vi "server 1.vi"() -> ()   [LabVIEW 2018]
doc: "This is the TCP server VI that supports multiple connections from client VIs."
uses:
  controls/TCP Multiple Connections State.ctl
  controls/TCP Multiple Connections Data.ctl
panel:
  out "Client IP":string
  out "color box":u32(colorbox)
  in  "Stop":bool
  out "Sent Data":dbl
  out "# of Connections":i32
  # "6341"
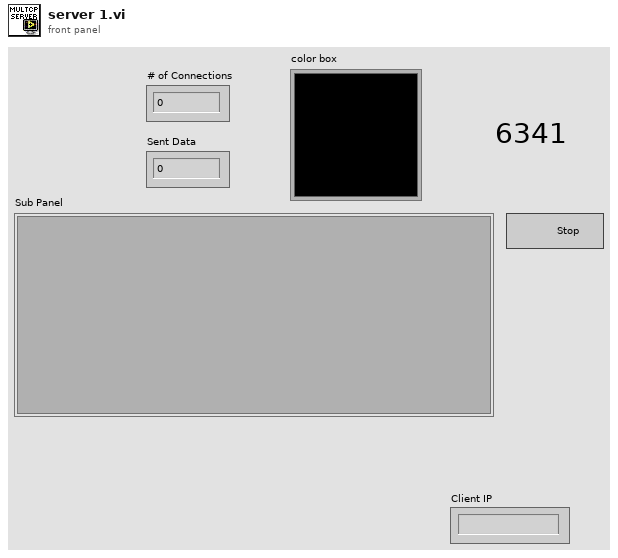
[diagram p1: front panel]
types:
  T1 = typedef "TCP Multiple Connections Data.ctl" = cluster{"Clients":refnum<k5>[], "Listener":refnum<k5>}
  T2 = typedef "TCP Multiple Connections State.ctl" = enum16{"Initialize", "Status Check", "Send Data", "Stop"}
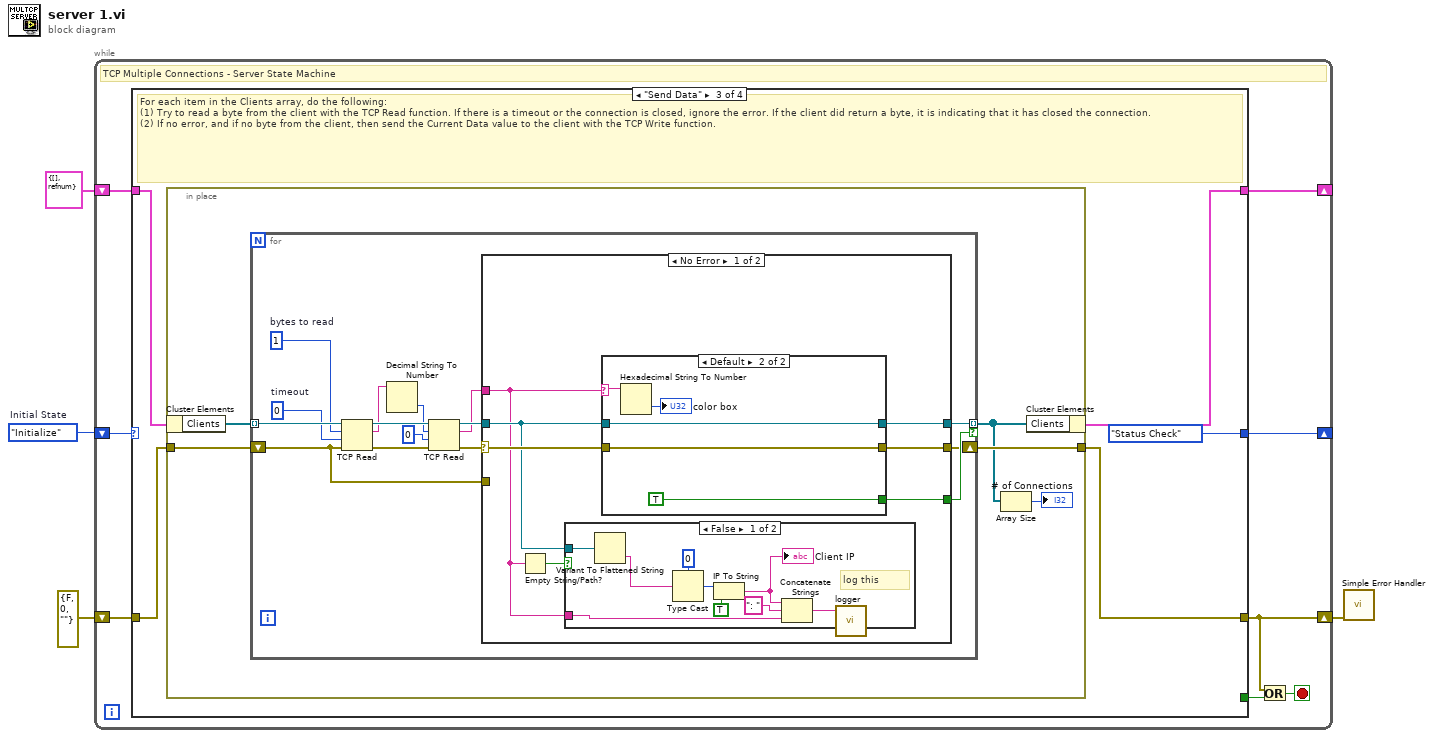
[diagram p0: block diagram]
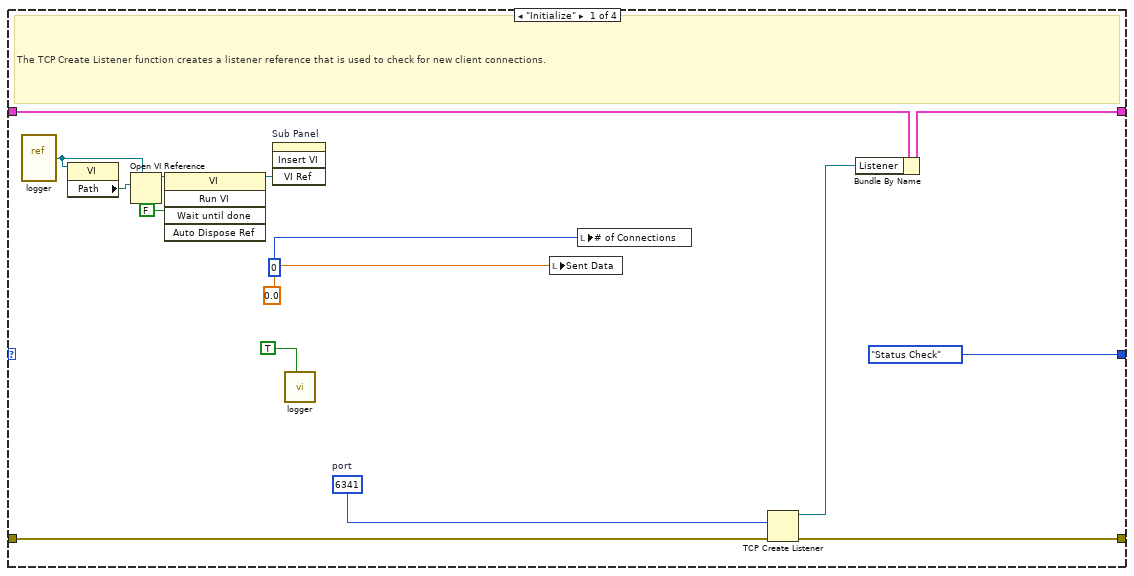
[diagram p2: hidden frame]
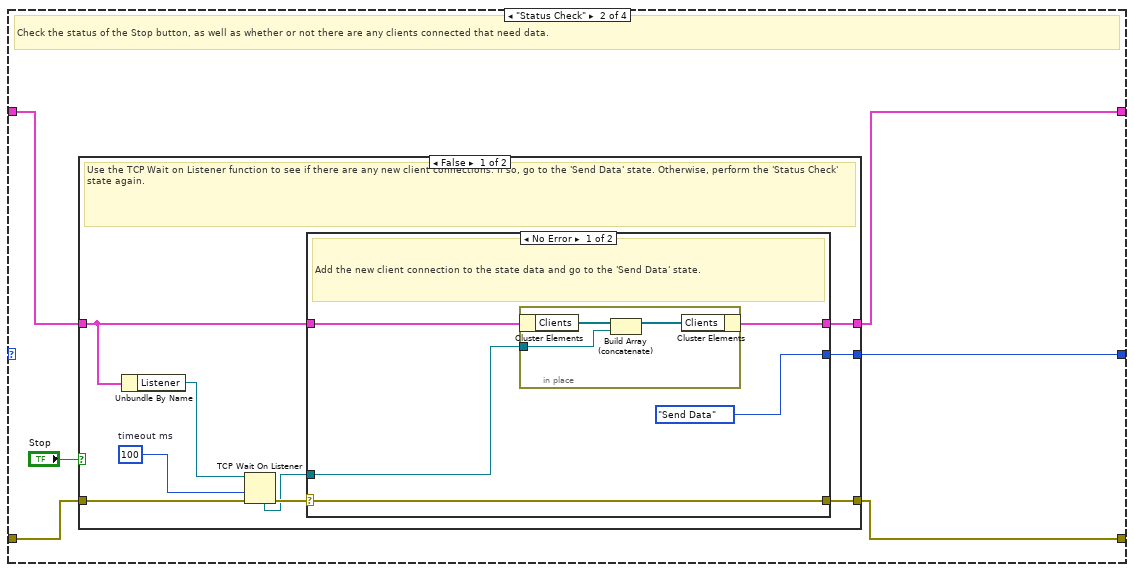
[diagram p3: hidden frame]
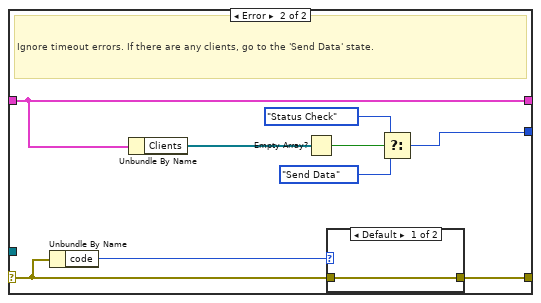
[diagram p4: hidden frame]
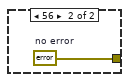
[diagram p5: hidden frame]
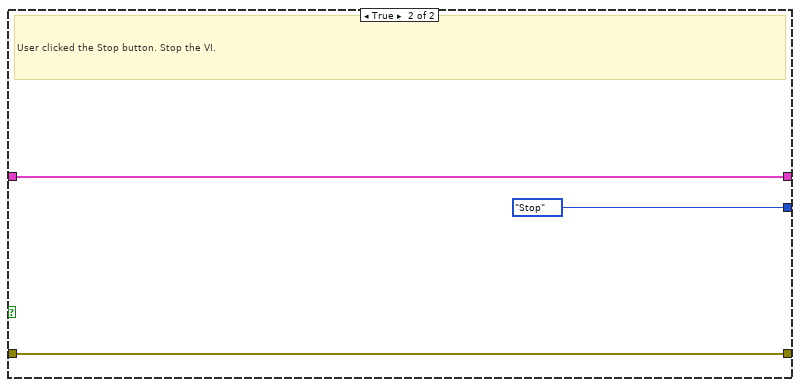
[diagram p6: hidden frame]
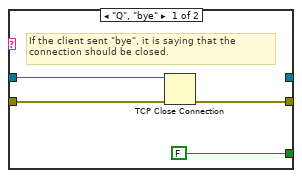
[diagram p8: hidden frame]
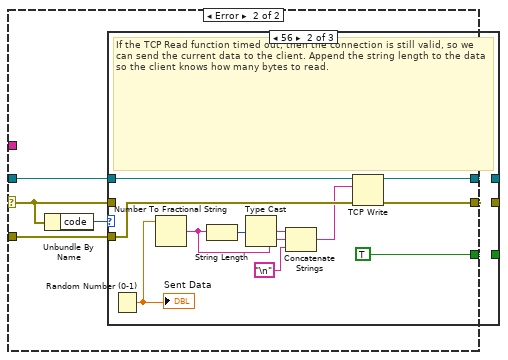
[diagram p9: hidden frame]
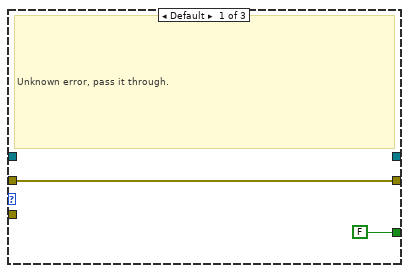
[diagram p10: hidden frame]
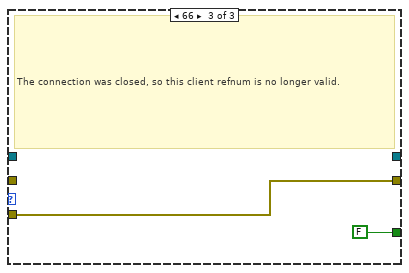
[diagram p11: hidden frame]
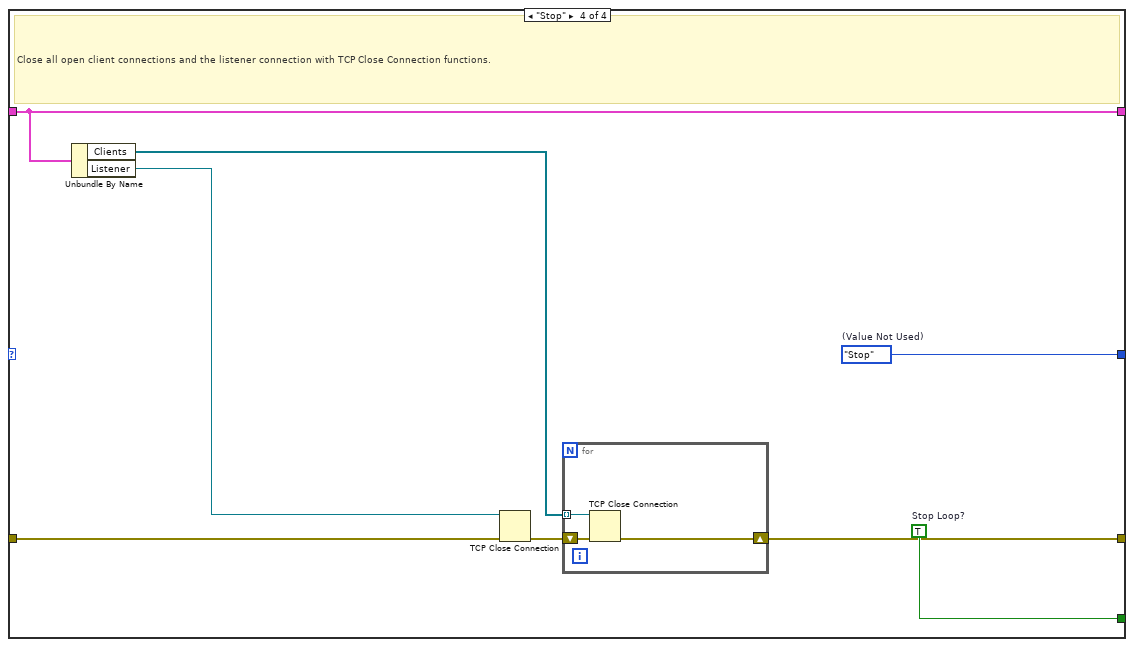
[diagram p12: hidden frame]
diagram:
  w4 = TCP_Multiple_Connections_State."Initialize"  # Initial State
  n1 = while {
    shift-right: [w11] -> _
    shift-left: w4 -> [w12]
    shift-right: [w9] -> _
    shift-left: T1 {"Clients"=[], "Listener"=refnum} ("Data") -> [w10]
    shift-right: [w5] -> w1
    shift-left: errorcluster {"status"=FALSE, "code"=0, "source"=""} ("error constant") -> [w8]
    stop <- w6 stop-if-true
    # "TCP Multiple Connections - Server State Machine"
    n2 = case shown="\"Send Data\"" w12 {
      tunnel: [TCP_Multiple_Connections_State."Status Check" ("States") w33 TCP_Multiple_Connections_State."Status Check" ("States") w137] -> w11
      tunnel: [_ _ _ w144] -> w7
      tunnel: w10 -> [w25 w31 w67 w143]
      tunnel: [w24 w30 w65 w143] -> w9
      tunnel: w8 -> [w27 w29 w69 w142]
      tunnel: [w26 w28 w68 w140] -> w5
      frame "Initialize" {
        w22 = u16 6341  # port
        # "The TCP Create Listener function creates a listener reference that is used to check for new client connections."
        n3 = vi-ref "logger.vi"() -> (w17:refnum<vi>)
        n4 = property class="VI"(reference=w17) -> ("Path"=w16:path)  [unwired: 1 in, 2 out]
        n5 = Open VI Reference(type specifier VI Refnum (for type only)=w17, vi path=w16) -> (vi reference=w15:refnum<vi>)  [unwired: 4 in, 1 out]
        n6 = invoke class="VI" method="Run VI"(reference=w15, "Wait until done"=FALSE ("Wait Until Done")) -> (reference out=w13:refnum<vi>)  [unwired: 3 in, 4 out]
        n7 = invoke on="Sub Panel" class="SubPnl" method="Insert VI"("VI Ref"=w13) -> ()  [unwired: 3 in, 4 out]
        n8 = call "logger.vi"("reset? (F)"=TRUE) -> ()  [unwired: 8 in, 1 out]
        n9 = local write "Sent Data"(0.0 ("Current Data")) -> ()
        n10 = local write "# of Connections"(0 ("Number of Client Connections")) -> ()
        n11 = TCP Create Listener(8:w27, 10:w22) -> (0:w26:errorcluster, 3:w23:refnum<k5>)  [unwired: 4 out]
        n12 = Bundle By Name(cluster=w25, "Listener"=w23) -> (w24:T1)
      }
      frame "Status Check" {
        # "Check the status of the Stop button, as well as whether or not there are any clients connected that need data."
        n13 = case shown="False" "Stop" {
          tunnel: [w42 TCP_Multiple_Connections_State."Stop" ("States")] -> w33
          tunnel: w29 -> [w41 w64]
          tunnel: [w34 w64] -> w28
          tunnel: w31 -> [w37 w63]
          tunnel: [w36 w63] -> w30
          frame False {
            w40 = 100  # timeout ms
            # "Use the TCP Wait on Listener function to see if there are any new client connections. If so, go to the 'Send Data' state. Otherwise, perform the 'Status Check' state again."
            n14 = Unbundle By Name(w37) -> ("Listener"=w35:refnum<k5>)
            n15 = TCP Wait On Listener(8:w41, 9:w40, 11:w35) -> (0:w39:errorcluster, 4:w38:refnum<k5>)  [unwired: 4 out]
            n16 = case shown="No Error" w39 {
              selector: w39 -> [w45 w59]
              tunnel: [TCP_Multiple_Connections_State."Send Data" ("States") w53] -> w42
              tunnel: w38 -> [w46 _]
              tunnel: w37 -> [w47 w56]
              tunnel: [w44 w56] -> w36
              tunnel: [w45 w57] -> w34
              frame No Error {
                # "Add the new client connection to the state data and go to the 'Send Data' state."
                n17 = in-place {
                  in-place-border: w46 -> [w48]
                  n18 = in-place-cluster #1(w47) -> ("Clients"=w50:refnum<k5>[])
                  n19 = Build Array (concatenate)(w50, w48) -> (w49:refnum<k5>[])
                  n20 = in-place-cluster #1("Clients"=w49) -> (w44:T1)
                }
              }
              frame Error {
                # "Ignore timeout errors. If there are any clients, go to the 'Send Data' state."
                n21 = Unbundle By Name(w59) -> ("code"=w58:i32)
                n22 = Unbundle By Name(w56) -> ("Clients"=w55:refnum<k5>[])
                n23 = Empty Array?(array=w55) -> (empty?=w54:bool)
                n24 = case shown="Default" w58 {
                  tunnel: w59 -> [w60 _]
                  tunnel: [w60 w61] -> w57
                  frame Default {
                  }
                  frame 56 {
                    w61 = errorcluster {"status"=FALSE, "code"=0, "source"=""}  # no error
                  }
                }
                n25 = Select(t=TCP_Multiple_Connections_State."Status Check" ("States"), s=w54, f=TCP_Multiple_Connections_State."Send Data" ("States")) -> (s? t:f=w53:T2)
              }
            }
          }
          frame True {
            # "User clicked the Stop button. Stop the VI."
          }
        }
      }
      frame "Send Data" {
        # "For each item in the Clients array, do the following:\n(1) Try to read a byte from the client with the TCP Read function. If there is a timeout or the connection is closed, ignore the error. If the client did return a byte, it is indicating that it has closed the connection.\n(2) If no error, and if no byte from the client, then send the Current Data value to the client with the TCP Write function."
        n26 = in-place {
          in-place-border: w69 -> [w74]
          in-place-border: [w73] -> w68
          n27 = in-place-cluster #2(w67) -> ("Clients"=w71:refnum<k5>[])
          n28 = for {
            tunnel: w71 -> [w89] mode=indexing
            shift-right: [w84] -> w73
            shift-left: w74 -> [w83]
            tunnel: [w86] -> w70 mode=indexing if=w85
            w87 = 0  # timeout
            w88 = 1  # bytes to read
            n29 = TCP Read(connection ID=w89, bytes to read=w88, error in (no error)=w83, 9:w87) -> (connection ID out=w82:refnum<k5>, data out=w80:string, error out=w78:errorcluster)  [unwired: 1 out]
            n30 = Decimal String To Number(string=w80) -> (number=w81:i32)  [unwired: 2 in, 1 out]
            n31 = TCP Read(connection ID=w82, bytes to read=w81, error in (no error)=w78, 9:0 ("timeout ms (25000)")) -> (connection ID out=w79:refnum<k5>, data out=w75:string, error out=w77:errorcluster)  [unwired: 1 out]
            n32 = case shown="No Error" w77 {
              selector: w77 -> [w96 w120]
              tunnel: w79 -> [w91 w117]
              tunnel: w75 -> [w90 _]
              tunnel: [w93 w115] -> w86
              tunnel: [w95 w116] -> w85
              tunnel: [w94 w119] -> w84
              tunnel: w83 -> [_ w118]
              frame No Error {
                # "If the client sent data, it is saying that the connection should be closed."
                n33 = Empty String/Path?(string/path=w90) -> (empty?=w92:bool)
                n34 = case shown="False" w92 {
                  tunnel: w91 -> [w98 _]
                  tunnel: w90 -> [w97 _]
                  frame False {
                    # "log this"
                    n35 = Variant To Flattened String(Variant=w98) -> (data string=w102:string)  [unwired: 1 out]
                    n36 = Type Cast(type=u32 0, x=w102) -> (*(type *) &x=w103:u32)
                    n37 = IP To String(1:TRUE ("dot notation? (F)"), 2:w103) -> (0:w104:string)
                    "Client IP" <- w104
                    n38 = Concatenate Strings(w104, ": " ("string"), w97) -> (w105:string)
                    n39 = call "logger.vi"("new data"=w105) -> ()  [unwired: 8 in, 1 out]
                  }
                  frame True {
                  }
                }
                n40 = case shown="Default" w90 {
                  selector: w90 -> [_ w112]
                  tunnel: w91 -> [w109 w110]
                  tunnel: w96 -> [w108 w114]
                  tunnel: [FALSE TRUE] -> w95
                  tunnel: [w106 w114] -> w94
                  tunnel: [_ w110] -> w93
                  frame "Q", "bye" {
                    # "If the client sent \"bye\", it is saying that the connection should be closed."
                    n41 = TCP Close Connection(connection ID=w109, error in (no error)=w108) -> (error out=w106:errorcluster)  [unwired: 2 out]
                  }
                  frame Default {
                    n42 = Hexadecimal String To Number(string=w112) -> (number=→"color box":u32)  [unwired: 2 in, 1 out]
                  }
                }
              }
              frame Error {
                # "Ignore connection closed and timeout errors"
                n43 = Unbundle By Name(w120) -> ("code"=w121:i32)
                n44 = case shown="56" w121 {
                  tunnel: w120 -> [w123 _ _]
                  tunnel: [w123 w134 w136] -> w119
                  tunnel: w118 -> [_ w130 w136]
                  tunnel: w117 -> [_ w133 _]
                  tunnel: [FALSE TRUE FALSE] -> w116
                  tunnel: [_ w132 _] -> w115
                  frame Default {
                    # "Unknown error, pass it through."
                  }
                  frame 56 {
                    # "If the TCP Read function timed out, then the connection is still valid, so we can send the current data to the client. Append the string length to the data so the client knows how many bytes to read."
                    n45 = Random Number (0-1)() -> (number: 0 to 1=w129:dbl)
                    "Sent Data" <- w129
                    n46 = Number To Fractional String(number=w129) -> (F-format string=w126:string)  [unwired: 3 in]
                    n47 = String Length(string=w126) -> (length=w127:i32)
                    n48 = Type Cast(x=w127) -> (*(type *) &x=w128:string)  [unwired: 1 in]
                    n49 = Concatenate Strings(w128, w126, "\n") -> (w125:string)
                    n50 = TCP Write(connection ID=w133, data in=w125, error in (no error)=w130) -> (connection ID out=w132:refnum<k5>, error out=w134:errorcluster)  [unwired: 2 out]
                  }
                  frame 66 {
                    # "The connection was closed, so this client refnum is no longer valid."
                  }
                }
              }
            }
          }
          n51 = Array Size(array=w70) -> (size(s)=→"# of Connections":i32)
          n52 = in-place-cluster #2("Clients"=w70) -> (w65:T1)
        }
      }
      frame "Stop" {
        w137 = TCP_Multiple_Connections_State."Stop"  # (Value Not Used)
        w144 = TRUE  # Stop Loop?
        # "Close all open client connections and the listener connection with TCP Close Connection functions."
        n53 = Unbundle By Name(w143) -> ("Clients"=w141:refnum<k5>[], "Listener"=w138:refnum<k5>)
        n54 = TCP Close Connection(connection ID=w138, error in (no error)=w142) -> (error out=w139:errorcluster)  [unwired: 1 in, 1 out]
        n55 = for {
          shift-right: [w146] -> w140
          shift-left: w139 -> [w147]
          tunnel: w141 -> [w145] mode=indexing
          n56 = TCP Close Connection(connection ID=w145, error in (no error)=w147) -> (error out=w146:errorcluster)  [unwired: 1 in, 1 out]
        }
      }
    }
    n57 = Or(x=w5, y=w7) -> (x .or. y?=w6:bool)
  }
  n58 = call <vilib>:"Simple Error Handler.vi"("error in (no error)"=w1) -> ()  [unwired: 4 in, 5 out]
